vi "GetLoopTunnelReference.vi"(8 "error in":errorcluster, 11 "LoopTunnel in":refnum<class "LoopTunnel.lvclass">) -> (0 "error out":errorcluster, 1 "reference out":refnum<vi>, 3 "LoopTunnel out":refnum<class "LoopTunnel.lvclass">)   [LabVIEW 2014, in "Raspberry Pi Compatible Compiler for LabVIEW.lvlib" / "LoopTunnel.lvclass"]
uses:
  LoopTunnel.lvclass
  Generic/Generic.lvclass
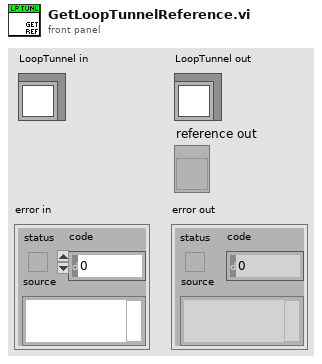
[diagram p1: front panel]
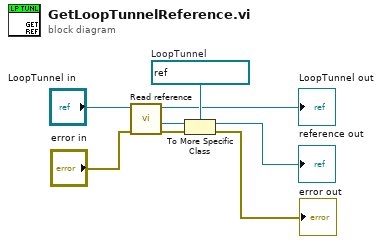
[diagram p0: block diagram]
diagram:
  w8 = refnum<vi> refnum  # LoopTunnel
  n1 = call "Read reference.vi"("error in"="error in", "GObject in"="LoopTunnel in") -> ("error out"=w7:errorcluster, "reference"=w6:refnum<vi>, "GObject out"=→"LoopTunnel out":refnum<class "LoopTunnel.lvclass">)  [unwired: 5 in]
  n2 = To More Specific Class(target class=w8, reference=w6, error in=w7) -> (specific class reference=→"reference out":refnum<vi>, error out=→"error out":errorcluster)
